vi "Paths Sub-Parser.vi"(2 "error in (no error)":errorcluster, 3 "Transformation Matrix":T1, 4 "Array of Nodes":string[](array[string])) -> (0 "error out":errorcluster, 1 "Path":T2(array[cluster]))   [LabVIEW 2013]
doc: "This VI parses paths found in an SVG file. It outputs colors, transformation matrices and organized arrays of commands used to specify each particular path."
uses:
  <vilib>/Analysis/Matrix/Datatypes/RealMatrix.ctl
  <vilib>/Analysis/baseanly.llb/Real A x B.vi
  <vilib>/Analysis/NI_AALBase.lvlib
  <vilib>/Analysis/Matrix/NI_Matrix.lvlib
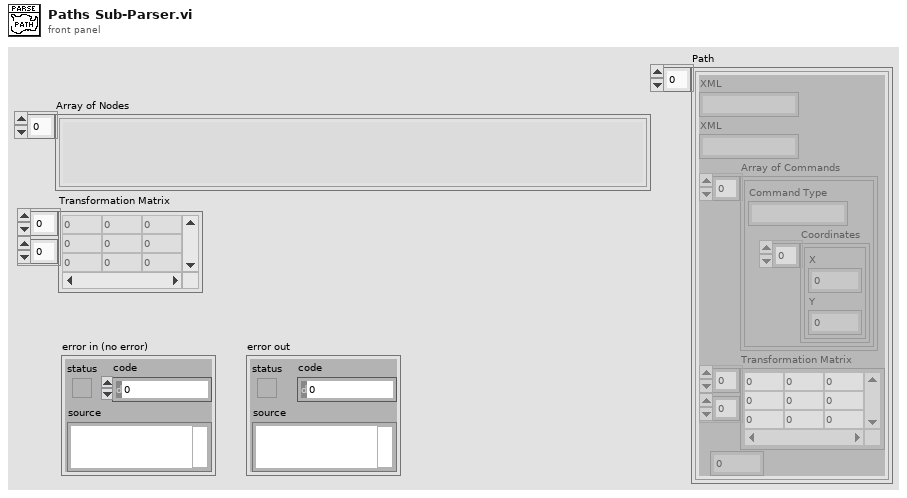
[diagram p1: front panel]
types:
  T1 = typedef "NI_Matrix.lvlib/RealMatrix.ctl" = dbl[][]
  T2 = cluster{"XML":string, "XML":string, "Array of Commands":cluster{"Command Type":string, "Coordinates":cluster{"X":dbl, "Y":dbl}[]}[], "Transformation Matrix":T1, "Order":i32}[]
  T3 = cluster{"XML":string, "XML":string, "Array of Commands":cluster{"Command Type":string, "Coordinates":cluster{"X":dbl, "Y":dbl}[]}[], "Transformation Matrix":T1, "Order":i32}
  T4 = cluster{"Command Type":string, "Coordinates":cluster{"X":dbl, "Y":dbl}[]}[]
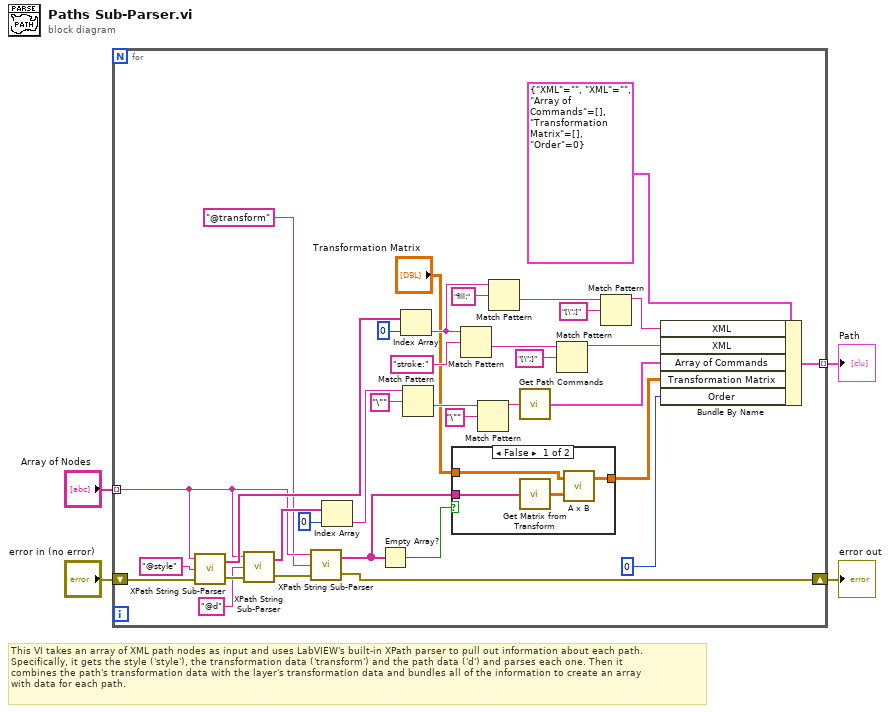
[diagram p0: block diagram]
diagram:
  # "This VI takes an array of XML path nodes as input and uses LabVIEW's built-in XPath parser to pull out information about each path. \nSpecifically, it gets the style ('style'), the transformation data ('transform') and the path data ('d') and parses each one. Then it\ncombines the path's transformation data with the layer's transformation data and bundles all of the information to create an array \nwith data for each path."
  n1 = for {
    tunnel: "Array of Nodes" -> [w12] mode=indexing
    shift-right: [w9] -> w2
    shift-left: "error in (no error)" -> [w32]
    tunnel: [w27] -> w1 mode=indexing
    n2 = call "XPath String Sub-Parser.vi"("error in (no error)"=w32, "XPath expression"="@style", "XML String"=w12) -> ("error out"=w24:errorcluster, "Array of Results"=w37:string[])
    n3 = call "XPath String Sub-Parser.vi"("error in (no error)"=w24, "XPath expression"="@d", "XML String"=w12) -> ("error out"=w10:errorcluster, "Array of Results"=w18:string[])
    n4 = call "XPath String Sub-Parser.vi"("error in (no error)"=w10, "XPath expression"="@transform", "XML String"=w12) -> ("error out"=w9:errorcluster, "Array of Results"=w14:string[])
    n5 = Index Array(array=w18, index=0) -> (element=w19:string)
    n6 = Empty Array?(array=w14) -> (empty?=w13:bool)
    n7 = Index Array(array=w37, index=0) -> (element=w29:string)
    n8 = Match Pattern(string=w19, regular expression="\"") -> (after substring=w21:string)  [unwired: 1 in, 3 out]
    n9 = case shown="False" w13 {
      tunnel: [w42 w43] -> w7
      tunnel: w14 -> [w40 _]
      tunnel: "Transformation Matrix" -> [w39 w43]
      frame False {
        n10 = call "Get Matrix from Transform.vi"("Transform Attributes"=w40) -> ("Matrix"=w41:T1)
        n11 = call-poly <vilib>:"A x B.vi"("B"=w41, "A"=w39) -> ("A x B"=w42:T1)  [unwired: 1 out]
      }
      frame True {
      }
    }
    n12 = Match Pattern(string=w29, regular expression="stroke:") -> (after substring=w30:string)  [unwired: 1 in, 3 out]
    n13 = Match Pattern(string=w21, regular expression="\"") -> (before substring=w16:string)  [unwired: 1 in, 3 out]
    n14 = Match Pattern(string=w29, regular expression="fill:") -> (after substring=w34:string)  [unwired: 1 in, 3 out]
    n15 = call "Get Path Commands.vi"("Commands Raw Data"=w16) -> ("Array of Commands"=w15:T4)
    n16 = Match Pattern(string=w30, regular expression="[\";]") -> (before substring=w25:string)  [unwired: 1 in, 3 out]
    n17 = Match Pattern(string=w34, regular expression="[\";]") -> (before substring=w26:string)  [unwired: 1 in, 3 out]
    n18 = Bundle By Name(cluster=T3 {"XML"="", "XML"="", "Array of Commands"=[], "Transformation Matrix"=[], "Order"=0} ("Cluster"), "XML"=w26, "XML"=w25, "Array of Commands"=w15, "Transformation Matrix"=w7, "Order"=0) -> (w27:T3)
  }
  "error out" <- w2
  "Path" <- w1
